vi "Get Buffer Actual Readings Count.vi"(0 "VISA resource name":refnum<visa-resource-name>, 5 "Timeout (10000 ms)":i32=10000 format="%#.6g", 7 "Buffer Name (defbuffer1)":string="defbuffer1", 11 "error in (no error)":errorcluster) -> (4 "VISA resource name out":refnum<visa-resource-name>, 6 "Actual Readings":i32, 15 "error out":errorcluster)   [LabVIEW 2023, in "Keithley DMM6500 DAQ6500 Series.lvlib"]
doc: "Returns the number of readings in the specified buffer."
uses:
  <instrlib>/Keithley DMM6500 DAQ6500 Series/Keithley DMM6500 DAQ6500 Series.lvlib
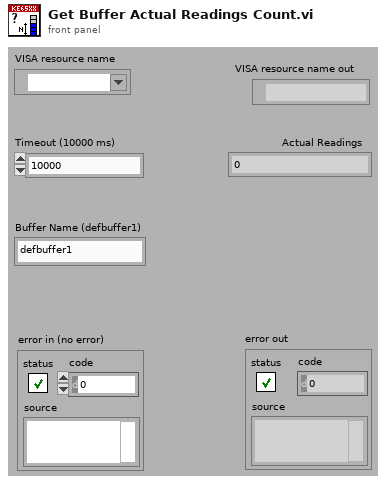
[diagram p1: front panel]
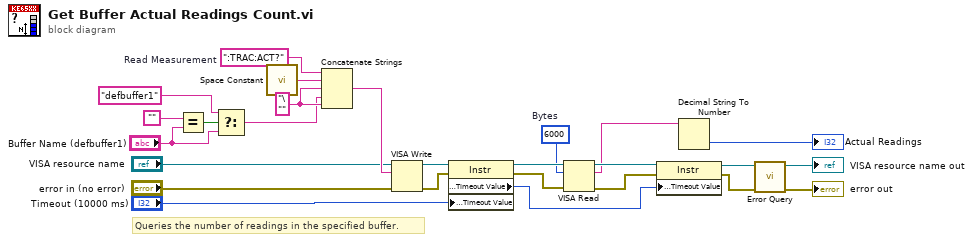
[diagram p0: block diagram]
diagram:
  w12 = "\""
  w9 = ":TRAC:ACT?"  # Read Measurement
  w18 = u32 6000  # Bytes
  # "Queries the number of readings in the specified buffer."
  n1 = Equal?(x="", y="Buffer Name (defbuffer1)") -> (x = y?=w15:bool)
  n2 = Select(t="defbuffer1", s=w15, f="Buffer Name (defbuffer1)") -> (s? t:f=w11:string)
  n3 = call <vilib>:"Space Constant.vi"() -> ("String"=w10:string)
  n4 = Concatenate Strings(w9, w10, w12, w11, w12) -> (w25:string)
  n5 = VISA Write(VISA resource name="VISA resource name", write buffer=w25, error in (no error)="error in (no error)") -> (VISA resource name out=w17:refnum<visa-resource-name>, error out=w24:errorcluster)  [unwired: 1 out]
  n6 = property class="Instr"(reference=w17, error in=w24, "General Settings:Timeout Value"="Timeout (10000 ms)") -> (reference out=w23:refnum<visa-resource-name>, error out=w22:errorcluster, "General Settings:Timeout Value"=w19:u32)
  n7 = VISA Read(VISA resource name=w23, byte count=w18, error in (no error)=w22) -> (VISA resource name out=w21:refnum<visa-resource-name>, read buffer=w2:string, error out=w20:errorcluster)  [unwired: 1 out]
  n8 = property class="Instr"(reference=w21, error in=w20, "General Settings:Timeout Value"=w19) -> (reference out=w4:refnum<visa-resource-name>, error out=w3:errorcluster)
  n9 = Decimal String To Number(string=w2) -> (number=→"Actual Readings":i32)  [unwired: 2 in, 1 out]
  n10 = call <instrlib>:"Error Query.vi"("error in (no error)"=w3, "VISA resource name"=w4) -> ("error out"=→"error out":errorcluster, "VISA resource name out"=→"VISA resource name out":refnum<visa-resource-name>)  [unwired: 6 in, 2 out]
